vi "KE6221 -- Set PDelta Power Meas Type.vi"(0 "6221 Resource In":refnum<visa-resource-name>, 1 "Check For SCPI Errors? (T)":bool=TRUE, 7 "Power Meas Type":T1, 11 "error in (no error)":errorcluster) -> (4 "6221 Resource Out (dupl)":refnum<visa-resource-name>, 15 "error out":errorcluster)   [LabVIEW 2019, in "Keithley 622x.lvlib"]
doc: "Sets the power measurement type that will be returned for 'Pulsed Delta' measurements (Average or Peak). This VI can only be used with a 6221 since the 6220 doesn't support 'Pulsed Delta' measurements. In addition, it is assumed that a 2182/2182A is connected to the 6221 to perform the acutal measurementss (i.e. the 6221 has no measurement capability)."
uses:
  Keithley 622x.lvlib
  Typedefs/KE6221 -- PDelta Power Meas Type.ctl
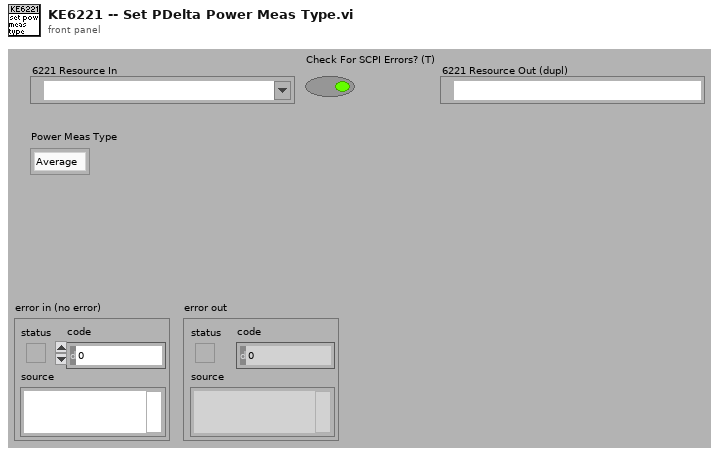
[diagram p1: front panel]
types:
  T1 = typedef "Keithley 622x.lvlib/KE6221 -- PDelta Power Meas Type.ctl" = enum16{"Average", "Peak"}
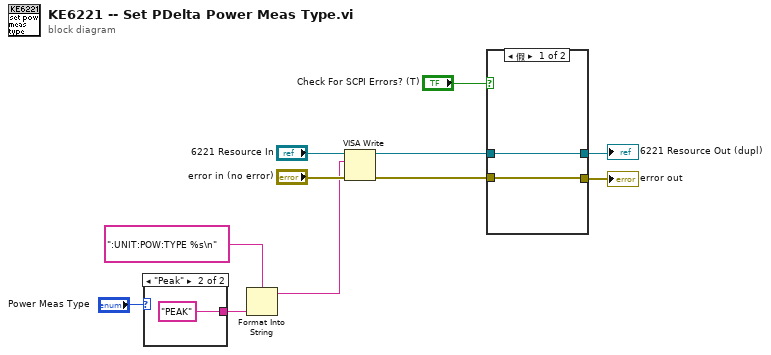
[diagram p0: block diagram]
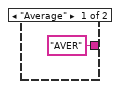
[diagram p2: hidden frame]
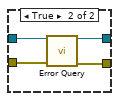
[diagram p3: hidden frame]
diagram:
  n1 = case shown="\"Peak\"" "Power Meas Type" {
    tunnel: ["AVER" "PEAK"] -> w4
    frame "Average" {
    }
    frame "Peak" {
    }
  }
  n2 = Format Into String(format string=":UNIT:POW:TYPE %s\n", w4) -> (resulting string=w3:string)  [unwired: 2 in, 1 out]
  n3 = VISA Write(VISA resource name="6221 Resource In", write buffer=w3, error in (no error)="error in (no error)") -> (VISA resource name out=w2:refnum<visa-resource-name>, error out=w1:errorcluster)  [unwired: 1 out]
  n4 = case shown="假" "Check For SCPI Errors? (T)" {
    tunnel: w2 -> [w15 w19]
    tunnel: w1 -> [w14 w18]
    tunnel: [w14 w17] -> w7
    tunnel: [w15 w16] -> w8
    frame False {
    }
    frame True {
      n5 = call "Error Query.vi"("VISA Resource In"=w19, "error in (no error)"=w18) -> ("VISA Resource Out (dupl)"=w16:refnum<visa-resource-name>, "error out"=w17:errorcluster)  [unwired: 10 in, 2 out]
    }
  }
  "6221 Resource Out (dupl)" <- w8
  "error out" <- w7
